vi "Write2TDMS.vi"(8 "Channel names":string[](array[string]), 9 "Group name":string, 10 "tdms file":refnum<k34>, 11 "Queue name":string) -> (2 "tdms file out":refnum<k34>, 3 "queue out":refnum<queue>)   [LabVIEW 2013]
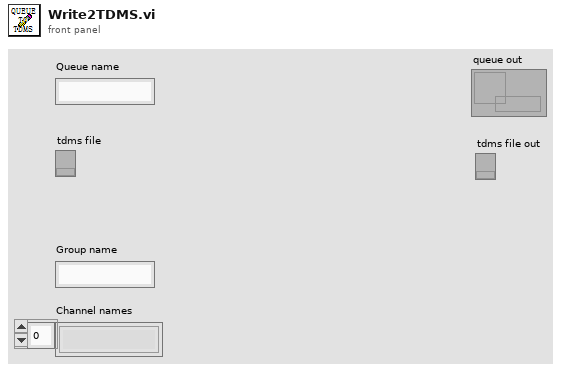
[diagram p1: front panel]
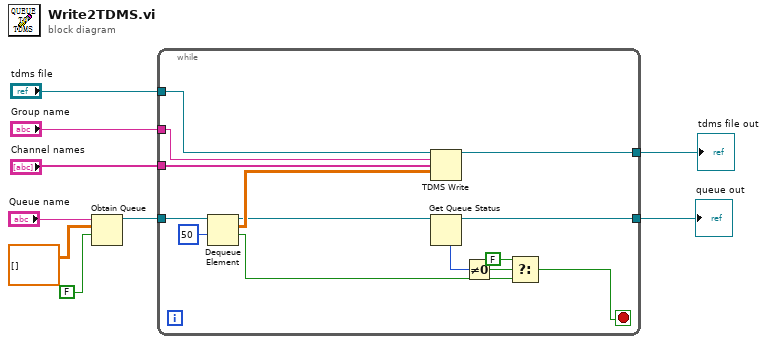
[diagram p0: block diagram]
diagram:
  n1 = Obtain Queue(name (unnamed)="Queue name", element data type=dbl[][] [], create if not found? (T)=FALSE) -> (queue out=w4:refnum<queue>)  [unwired: 2 in, 2 out]
  n2 = while {
    tunnel: "tdms file" -> [w23]
    tunnel: "Group name" -> [w22]
    tunnel: "Channel names" -> [w21]
    tunnel: w4 -> [w20]
    tunnel: [w17] -> w3
    tunnel: [w10] -> w1
    stop <- w13 stop-if-true
    n3 = Dequeue Element(queue=w20, timeout in ms (-1)=50) -> (queue out=w18:refnum<queue>, element=w19:dbl[][], timed out?=w11:bool)  [unwired: 1 in, 1 out]
    n4 = TDMS Write(0:w23, 5:w22, 7:w21, 9:w19) -> (4:w10:refnum<k34>)  [unwired: 2 in, 3 out]
    n5 = Get Queue Status(queue=w18) -> (queue out=w17:refnum<queue>, # elements in queue=w14:i32)  [unwired: 2 in, 6 out]
    n6 = Not Equal To 0?(x=w14) -> (x != 0?=w15:bool)
    n7 = Select(t=FALSE, s=w15, f=w11) -> (s? t:f=w13:bool)
  }
  "queue out" <- w3
  "tdms file out" <- w1
